vi "LVObject to JSON.vi"(5 "enable LabVIEW extensions? (T)":bool=TRUE, 6 "Pretty Print?":bool, 7 "Class 1 in":refnum<class "Serializer-Scheme.lvclass">, 8 "error in":errorcluster, 10 "Object":refnum<class>) -> (0 "error out":errorcluster, 2 "<JSON>Object":string)   [LabVIEW 2021, in "TSC Material Theme.lvlib" / "Serializer-Scheme.lvclass"]
doc: "Convert Object of a LabVIEW Class to a JSON representation."
uses:
  Serializer-Scheme.lvclass
  TSC Material Theme/material json scheme--cluster.ctl
  Material-Scheme/Material-Scheme.lvclass
  Material-Scheme/Material-Scheme.lvclass/Material-Scheme.ctl
  Material-Scheme/data member access/Get primary.vi
  Material-Scheme/data member access/Get surfaceTint.vi
  Material-Scheme/data member access/Get onPrimary.vi
  Material-Scheme/data member access/Get primaryContainer.vi
  Material-Scheme/data member access/Get onPrimaryContainer.vi
  Material-Scheme/data member access/Get secondary.vi
  Material-Scheme/data member access/Get onSecondary.vi
  Material-Scheme/data member access/Get secondaryContainer.vi
  Material-Scheme/data member access/Get onSecondaryContainer.vi
  Material-Scheme/data member access/Get tertiary.vi
  Material-Scheme/data member access/Get onTertiary.vi
  Material-Scheme/data member access/Get tertiaryContainer.vi
  Material-Scheme/data member access/Get onTertiaryContainer.vi
  Material-Scheme/data member access/Get error.vi
  Material-Scheme/data member access/Get onError.vi
  Material-Scheme/data member access/Get errorContainer.vi
  Material-Scheme/data member access/Get onErrorContainer.vi
  Material-Scheme/data member access/get background.vi
  Material-Scheme/data member access/Get onBackground.vi
  Material-Scheme/data member access/get surface.vi
  Material-Scheme/data member access/Get onSurface.vi
  Material-Scheme/data member access/get surfaceVariant.vi
  Material-Scheme/data member access/Get onSurfaceVariant.vi
  Material-Scheme/data member access/Get outline.vi
  Material-Scheme/data member access/Get outlineVariant.vi
  Material-Scheme/data member access/Get shadow.vi
  Material-Scheme/data member access/Get scrim.vi
  Material-Scheme/data member access/get inverseSurface.vi
  Material-Scheme/data member access/Get inverseOnSurface.vi
  Material-Scheme/data member access/Get inversePrimary.vi
  Material-Scheme/data member access/Get primaryFixed.vi
  Material-Scheme/data member access/Get onPrimaryFixed.vi
  Material-Scheme/data member access/Get primaryFixedDim.vi
  Material-Scheme/data member access/Get onPrimaryFixedVariant.vi
  Material-Scheme/data member access/Get secondaryFixed.vi
  Material-Scheme/data member access/Get onSecondaryFixed.vi
  Material-Scheme/data member access/Get secondaryFixedDim.vi
  Material-Scheme/data member access/Get onSecondaryFixedVariant.vi
  Material-Scheme/data member access/Get tertiaryFixed.vi
  Material-Scheme/data member access/Get onTertiaryFixed.vi
  Material-Scheme/data member access/Get tertiaryFixedDim.vi
  Material-Scheme/data member access/Get onTertiaryFixedVariant.vi
  Material-Scheme/data member access/get surfaceDim.vi
  Material-Scheme/data member access/get surfaceBright.vi
  Material-Scheme/data member access/get surfaceContainerLowest.vi
  Material-Scheme/data member access/get surfaceContainerLow.vi
  Material-Scheme/data member access/get surfaceContainer.vi
  Material-Scheme/data member access/get surfaceContainerHigh.vi
  Material-Scheme/data member access/get surfaceContainerHighest.vi
  TSC Material Theme/TSC Material Theme.lvlib
  <vilib>/JDP Science/JSONtext/JSONtext.lvlib
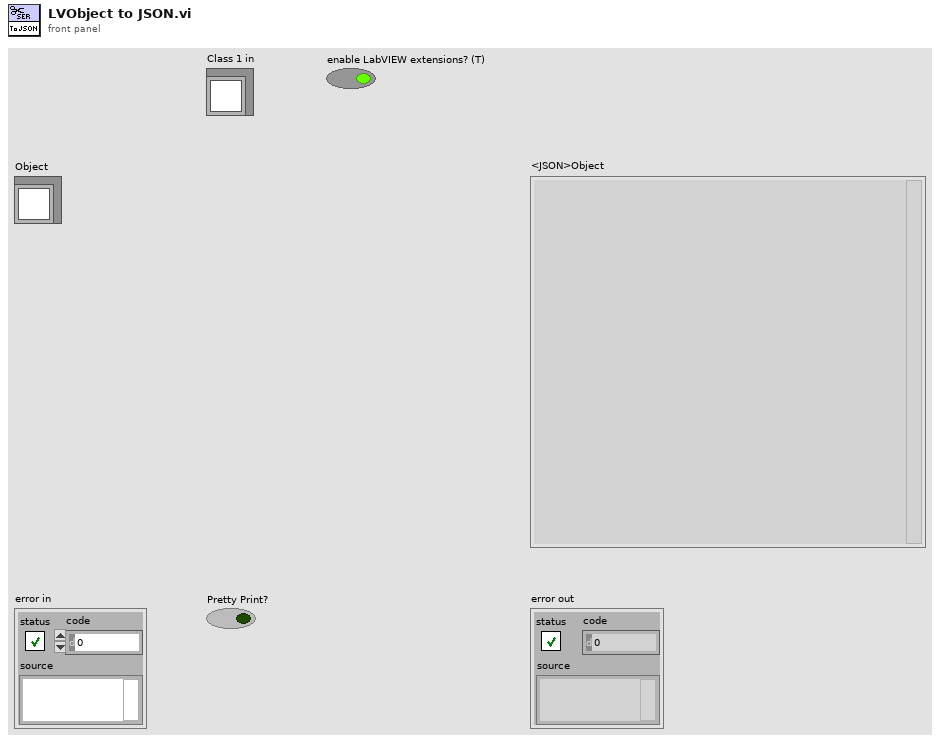
[diagram p1: front panel]
types:
  T1 = typedef "TSC Material Theme.lvlib/material json scheme--cluster.ctl" = cluster{"primary":string, "surfaceTint":string, "onPrimary":string, "primaryContainer":string, "onPrimaryContainer":string, "secondary":string, "onSecondary":string, "secondaryContainer":string, "onSecondaryContainer":string, "tertiary":string, "onTertiary":string, "tertiaryContainer":string, "onTertiaryContainer":string, "error":string, "onError":string, "errorContainer":string, "onErrorContainer":string, "background":string, "onBackground":string, "surface":string, "onSurface":string, "surfaceVariant":string, "onSurfaceVariant":string, "outline":string, "outlineVariant":string, "shadow":string, "scrim":string, "inverseSurface":string, "inverseOnSurface":string, "inversePrimary":string, "primaryFixed":string, "onPrimaryFixed":string, "primaryFixedDim":string, "onPrimaryFixedVariant":string, "secondaryFixed":string, "onSecondaryFixed":string, "secondaryFixedDim":string, "onSecondaryFixedVariant":string, "tertiaryFixed":string, "onTertiaryFixed":string, "tertiaryFixedDim":string, "onTertiaryFixedVariant":string, "surfaceDim":string, "surfaceBright":string, "surfaceContainerLowest":string, "surfaceContainerLow":string, "surfaceContainer":string, "surfaceContainerHigh":string, "surfaceContainerHighest":string}
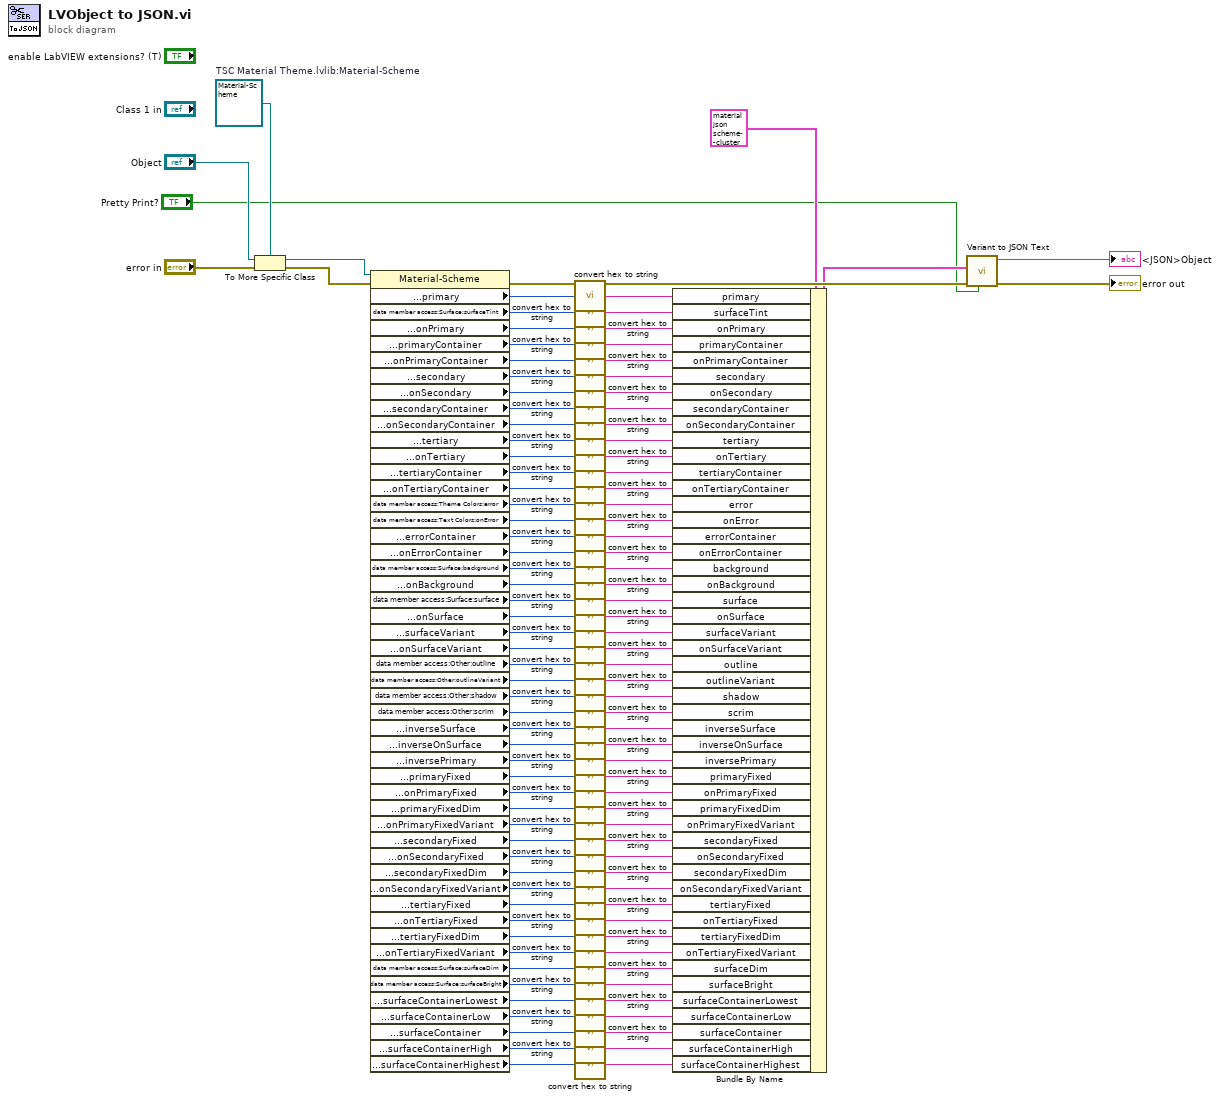
[diagram p0: block diagram]
diagram:
  w104 = refnum<class "Material-Scheme.lvclass"> refnum  # TSC Material Theme.lvlib:Material-Scheme
  n1 = To More Specific Class(target class=w104, reference="Object", error in="error in") -> (specific class reference=w4:refnum<class "Material-Scheme.lvclass">, error out=w108:errorcluster)
  n2 = property class="Material-Scheme"(reference=w4, error in=w108) -> (error out=w106:errorcluster, "data member access:Theme Colors:primary"=w103:u32, "data member access:Surface:surfaceTint"=w100:u32, "data member access:Text Colors:onPrimary"=w83:u32, "data member access:Theme Colors:primaryContainer"=w82:u32, "data member access:Text Colors:onPrimaryContainer"=w81:u32, "data member access:Theme Colors:secondary"=w80:u32, "data member access:Text Colors:onSecondary"=w79:u32, "data member access:Theme Colors:secondaryContainer"=w78:u32, "data member access:Text Colors:onSecondaryContainer"=w77:u32, "data member access:Theme Colors:tertiary"=w76:u32, "data member access:Text Colors:onTertiary"=w75:u32, "data member access:Theme Colors:tertiaryContainer"=w74:u32, "data member access:Text Colors:onTertiaryContainer"=w73:u32, "data member access:Theme Colors:error"=w72:u32, "data member access:Text Colors:onError"=w71:u32, "data member access:Theme Colors:errorContainer"=w70:u32, "data member access:Text Colors:onErrorContainer"=w69:u32, "data member access:Surface:background"=w68:u32, "data member access:Text Colors:onBackground"=w49:u32, "data member access:Surface:surface"=w48:u32, "data member access:Text Colors:onSurface"=w47:u32, "data member access:Surface:surfaceVariant"=w46:u32, "data member access:Text Colors:onSurfaceVariant"=w45:u32, "data member access:Other:outline"=w44:u32, "data member access:Other:outlineVariant"=w43:u32, "data member access:Other:shadow"=w42:u32, "data member access:Other:scrim"=w41:u32, "data member access:Surface:inverseSurface"=w40:u32, "data member access:Text Colors:inverseOnSurface"=w39:u32, "data member access:Theme Colors:inversePrimary"=w38:u32, "data member access:Fixed Colors:primaryFixed"=w37:u32, "data member access:Text Colors Fixed:onPrimaryFixed"=w36:u32, "data member access:Fixed Colors:primaryFixedDim"=w35:u32, "data member access:Text Colors Fixed:onPrimaryFixedVariant"=w34:u32, "data member access:Fixed Colors:secondaryFixed"=w33:u32, "data member access:Text Colors Fixed:onSecondaryFixed"=w32:u32, "data member access:Fixed Colors:secondaryFixedDim"=w30:u32, "data member access:Text Colors Fixed:onSecondaryFixedVariant"=w29:u32, "data member access:Fixed Colors:tertiaryFixed"=w28:u32, "data member access:Text Colors Fixed:onTertiaryFixed"=w27:u32, "data member access:Fixed Colors:tertiaryFixedDim"=w26:u32, "data member access:Text Colors Fixed:onTertiaryFixedVariant"=w25:u32, "data member access:Surface:surfaceDim"=w24:u32, "data member access:Surface:surfaceBright"=w23:u32, "data member access:Surface:surfaceContainerLowest"=w22:u32, "data member access:Surface:surfaceContainerLow"=w21:u32, "data member access:Surface:surfaceContainer"=w6:u32, "data member access:Surface:surfaceContainerHigh"=w7:u32, "data member access:Surface:surfaceContainerHighest"=w8:u32)  [unwired: 1 out]
  n3 = call "convert hex to string.vi"("hex"=w103) -> ("string"=w102:string)
  n4 = call "convert hex to string.vi"("hex"=w100) -> ("string"=w101:string)
  n5 = call "convert hex to string.vi"("hex"=w83) -> ("string"=w99:string)
  n6 = call "convert hex to string.vi"("hex"=w82) -> ("string"=w98:string)
  n7 = call "convert hex to string.vi"("hex"=w81) -> ("string"=w97:string)
  n8 = call "convert hex to string.vi"("hex"=w80) -> ("string"=w96:string)
  n9 = call "convert hex to string.vi"("hex"=w79) -> ("string"=w95:string)
  n10 = call "convert hex to string.vi"("hex"=w78) -> ("string"=w94:string)
  n11 = call "convert hex to string.vi"("hex"=w77) -> ("string"=w93:string)
  n12 = call "convert hex to string.vi"("hex"=w76) -> ("string"=w92:string)
  n13 = call "convert hex to string.vi"("hex"=w75) -> ("string"=w91:string)
  n14 = call "convert hex to string.vi"("hex"=w74) -> ("string"=w90:string)
  n15 = call "convert hex to string.vi"("hex"=w73) -> ("string"=w89:string)
  n16 = call "convert hex to string.vi"("hex"=w72) -> ("string"=w88:string)
  n17 = call "convert hex to string.vi"("hex"=w71) -> ("string"=w87:string)
  n18 = call "convert hex to string.vi"("hex"=w70) -> ("string"=w86:string)
  n19 = call "convert hex to string.vi"("hex"=w69) -> ("string"=w85:string)
  n20 = call "convert hex to string.vi"("hex"=w68) -> ("string"=w84:string)
  n21 = call "convert hex to string.vi"("hex"=w49) -> ("string"=w67:string)
  n22 = call "convert hex to string.vi"("hex"=w48) -> ("string"=w66:string)
  n23 = call "convert hex to string.vi"("hex"=w47) -> ("string"=w65:string)
  n24 = call "convert hex to string.vi"("hex"=w46) -> ("string"=w64:string)
  n25 = call "convert hex to string.vi"("hex"=w45) -> ("string"=w63:string)
  n26 = call "convert hex to string.vi"("hex"=w44) -> ("string"=w62:string)
  n27 = call "convert hex to string.vi"("hex"=w43) -> ("string"=w61:string)
  n28 = call "convert hex to string.vi"("hex"=w42) -> ("string"=w60:string)
  n29 = call "convert hex to string.vi"("hex"=w41) -> ("string"=w59:string)
  n30 = call "convert hex to string.vi"("hex"=w40) -> ("string"=w58:string)
  n31 = call "convert hex to string.vi"("hex"=w39) -> ("string"=w57:string)
  n32 = call "convert hex to string.vi"("hex"=w38) -> ("string"=w56:string)
  n33 = call "convert hex to string.vi"("hex"=w37) -> ("string"=w55:string)
  n34 = call "convert hex to string.vi"("hex"=w36) -> ("string"=w54:string)
  n35 = call "convert hex to string.vi"("hex"=w35) -> ("string"=w53:string)
  n36 = call "convert hex to string.vi"("hex"=w34) -> ("string"=w52:string)
  n37 = call "convert hex to string.vi"("hex"=w33) -> ("string"=w51:string)
  n38 = call "convert hex to string.vi"("hex"=w32) -> ("string"=w50:string)
  n39 = call "convert hex to string.vi"("hex"=w30) -> ("string"=w31:string)
  n40 = call "convert hex to string.vi"("hex"=w29) -> ("string"=w13:string)
  n41 = call "convert hex to string.vi"("hex"=w28) -> ("string"=w12:string)
  n42 = call "convert hex to string.vi"("hex"=w27) -> ("string"=w14:string)
  n43 = call "convert hex to string.vi"("hex"=w26) -> ("string"=w15:string)
  n44 = call "convert hex to string.vi"("hex"=w25) -> ("string"=w16:string)
  n45 = call "convert hex to string.vi"("hex"=w24) -> ("string"=w17:string)
  n46 = call "convert hex to string.vi"("hex"=w23) -> ("string"=w18:string)
  n47 = call "convert hex to string.vi"("hex"=w22) -> ("string"=w19:string)
  n48 = call "convert hex to string.vi"("hex"=w21) -> ("string"=w20:string)
  n49 = call "convert hex to string.vi"("hex"=w6) -> ("string"=w11:string)
  n50 = call "convert hex to string.vi"("hex"=w7) -> ("string"=w10:string)
  n51 = call "convert hex to string.vi"("hex"=w8) -> ("string"=w9:string)
  n52 = Bundle By Name(cluster=T1 {"primary"="", "surfaceTint"="", "onPrimary"="", "primaryContainer"="", "onPrimaryContainer"="", "secondary"="", "onSecondary"="", "secondaryContainer"="", "onSecondaryContainer"="", "tertiary"="", "onTertiary"="", "tertiaryContainer"="", "onTertiaryContainer"="", "error"="", "onError"="", "errorContainer"="", "onErrorContainer"="", "background"="", "onBackground"="", "surface"="", "onSurface"="", "surfaceVariant"="", "onSurfaceVariant"="", "outline"="", "outlineVariant"="", "shadow"="", "scrim"="", "inverseSurface"="", "inverseOnSurface"="", "inversePrimary"="", "primaryFixed"="", "onPrimaryFixed"="", "primaryFixedDim"="", "onPrimaryFixedVariant"="", "secondaryFixed"="", "onSecondaryFixed"="", "secondaryFixedDim"="", "onSecondaryFixedVariant"="", "tertiaryFixed"="", "onTertiaryFixed"="", "tertiaryFixedDim"="", "onTertiaryFixedVariant"="", "surfaceDim"="", "surfaceBright"="", "surfaceContainerLowest"="", "surfaceContainerLow"="", "surfaceContainer"="", "surfaceContainerHigh"="", "surfaceContainerHighest"=""} ("light"), "primary"=w102, "surfaceTint"=w101, "onPrimary"=w99, "primaryContainer"=w98, "onPrimaryContainer"=w97, "secondary"=w96, "onSecondary"=w95, "secondaryContainer"=w94, "onSecondaryContainer"=w93, "tertiary"=w92, "onTertiary"=w91, "tertiaryContainer"=w90, "onTertiaryContainer"=w89, "error"=w88, "onError"=w87, "errorContainer"=w86, "onErrorContainer"=w85, "background"=w84, "onBackground"=w67, "surface"=w66, "onSurface"=w65, "surfaceVariant"=w64, "onSurfaceVariant"=w63, "outline"=w62, "outlineVariant"=w61, "shadow"=w60, "scrim"=w59, "inverseSurface"=w58, "inverseOnSurface"=w57, "inversePrimary"=w56, "primaryFixed"=w55, "onPrimaryFixed"=w54, "primaryFixedDim"=w53, "onPrimaryFixedVariant"=w52, "secondaryFixed"=w51, "onSecondaryFixed"=w50, "secondaryFixedDim"=w31, "onSecondaryFixedVariant"=w13, "tertiaryFixed"=w12, "onTertiaryFixed"=w14, "tertiaryFixedDim"=w15, "onTertiaryFixedVariant"=w16, "surfaceDim"=w17, "surfaceBright"=w18, "surfaceContainerLowest"=w19, "surfaceContainerLow"=w20, "surfaceContainer"=w11, "surfaceContainerHigh"=w10, "surfaceContainerHighest"=w9) -> (w3:T1)
  n53 = call <vilib>:"Variant to JSON Text.vi"("Pretty Print?"="Pretty Print?", "error in (no error)"=w106, "Variant"=w3) -> ("error out"=→"error out":errorcluster, "<JSON>"=→"<JSON>Object":string)  [unwired: 6 in, 1 out]
